vi "ForLoopExample_Array.vi"() -> ()   [LabVIEW 2020]
panel:
  out "Tablica 2":dbl[](array[numeric])
  in  "Tablica 1":dbl[](array[numeric])
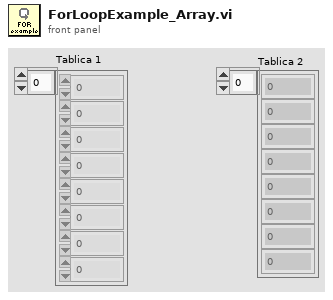
[diagram p1: front panel]
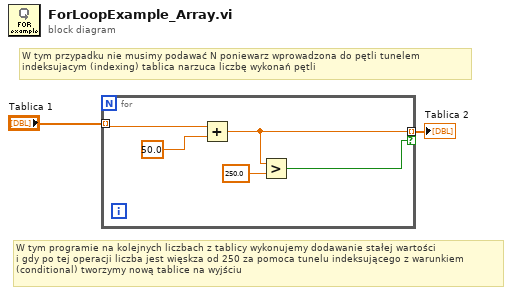
[diagram p0: block diagram]
diagram:
  # "W tym programie na kolejnych liczbach z tablicy wykonujemy dodawanie stałej wartości\ni gdy po tej operacji liczba jest więskza od 250 za pomoca tunelu indeksującego z warunkiem\n(conditional) tworzymy nową tablice na wyjściu"
  # "W tym przypadku nie musimy podawać N poniewarz wprowadzona do pętli tunelem \nindeksujacym (indexing) tablica narzuca liczbę wykonań pętli"
  n1 = for {
    tunnel: "Tablica 1" -> [w7] mode=indexing
    tunnel: [w4] -> w1 mode=indexing if=w3
    n2 = Add(x=w7, y=50.0) -> (x+y=w4:dbl)
    n3 = Greater?(x=w4, y=250.0) -> (0:w3:bool)
  }
  "Tablica 2" <- w1
